vi "ziUpdateDevice.vi"(10 "file path (use dialog)":path=path "Z:/ziReleases/ci-artifacts/trunk/r49020-2017-11-30_15-47-53/LabOneMF-17.12.49020.tar", 11 "Address":string="DEV") -> (0 "Error Out":errorcluster)   [LabVIEW 2009, in "Zurich Instruments LabOne.lvlib"]
doc: "Allow to Update MFLI/UHF devices via the Labview API.\nNOTE: \nDO NOT TURN OFF POWER OR UNPLUG THE DEVICE FROM YOUR SYSTEM.PLEASE, WAIT UNTIL THE DEVICE IS FINISHED."
uses:
  <instrlib>/Zurich Instruments LabOne/Zurich Instruments LabOne.lvlib
  <instrlib>/Zurich Instruments LabOne/Public/Configure/ziGetValueString.vi
  <instrlib>/Zurich Instruments LabOne/Public/Configure/ziSetValueDouble.vi
  <instrlib>/Zurich Instruments LabOne/Public/Data/ziTypeCoreVectorWave.ctl
  <instrlib>/Zurich Instruments LabOne/Public/Configure/ziSetVector.vi
  <instrlib>/Zurich Instruments LabOne/Private/ziLV32.dll
panel:
  # "NOTE: \nDO NOT TURN OFF POWER OR UNPLUG \nTHE DEVICE FROM YOUR SYSTEM.\nPLEASE, WAIT UNTIL THE DEVICE IS FINISHED."
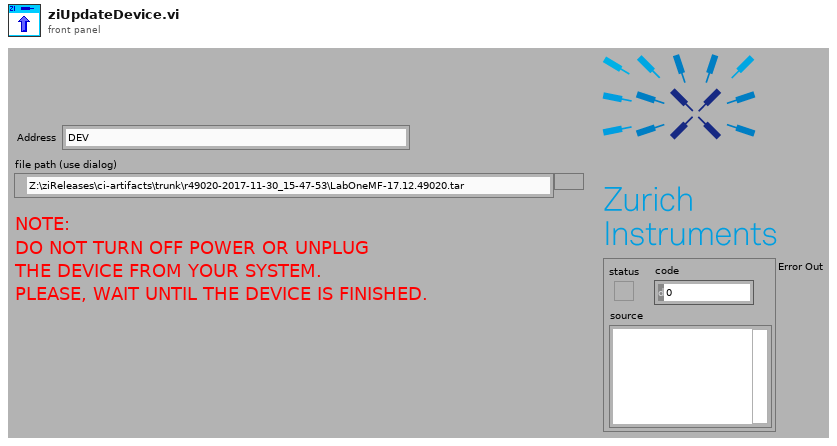
[diagram p1: front panel]
types:
  T1 = typedef "Zurich Instruments LabOne.lvlib/ziTypeCoreVectorWave.ctl" = cluster{"Timestamp (ticks)":u64, "Sequence Number":u32, "total Elements":u64, "Block Offset":u64, "Block Elements":u32, "Flags":u8, "Element Type":u8, "Data UInt8":u8[], "Data UInt16":u16[], "Data UInt32":u32[], "Data UInt64":u64[], "Data Float":sgl[], "Data Double":dbl[], "Data String":string}
  T2 = typedef "Zurich Instruments LabOne.lvlib/ziTypeHandle.ctl" = cluster{"handleValid":bool, "Conn":u64, "Path Prefix":string, "Handle":u64, "Connected":bool, "Clockbase(s)":dbl}
  T3 = typedef "ziTypeDisovery.ctl" = cluster{"timestamp":u64, "deviceid":string, "devicetype":string, "serveraddress":string, "serverport":u32, "apilevel":u32, "discoverable":bool, "interface":string, "connected":string, "available":bool, "owner":string, "status":string, "options ":string, "serverversion":string}
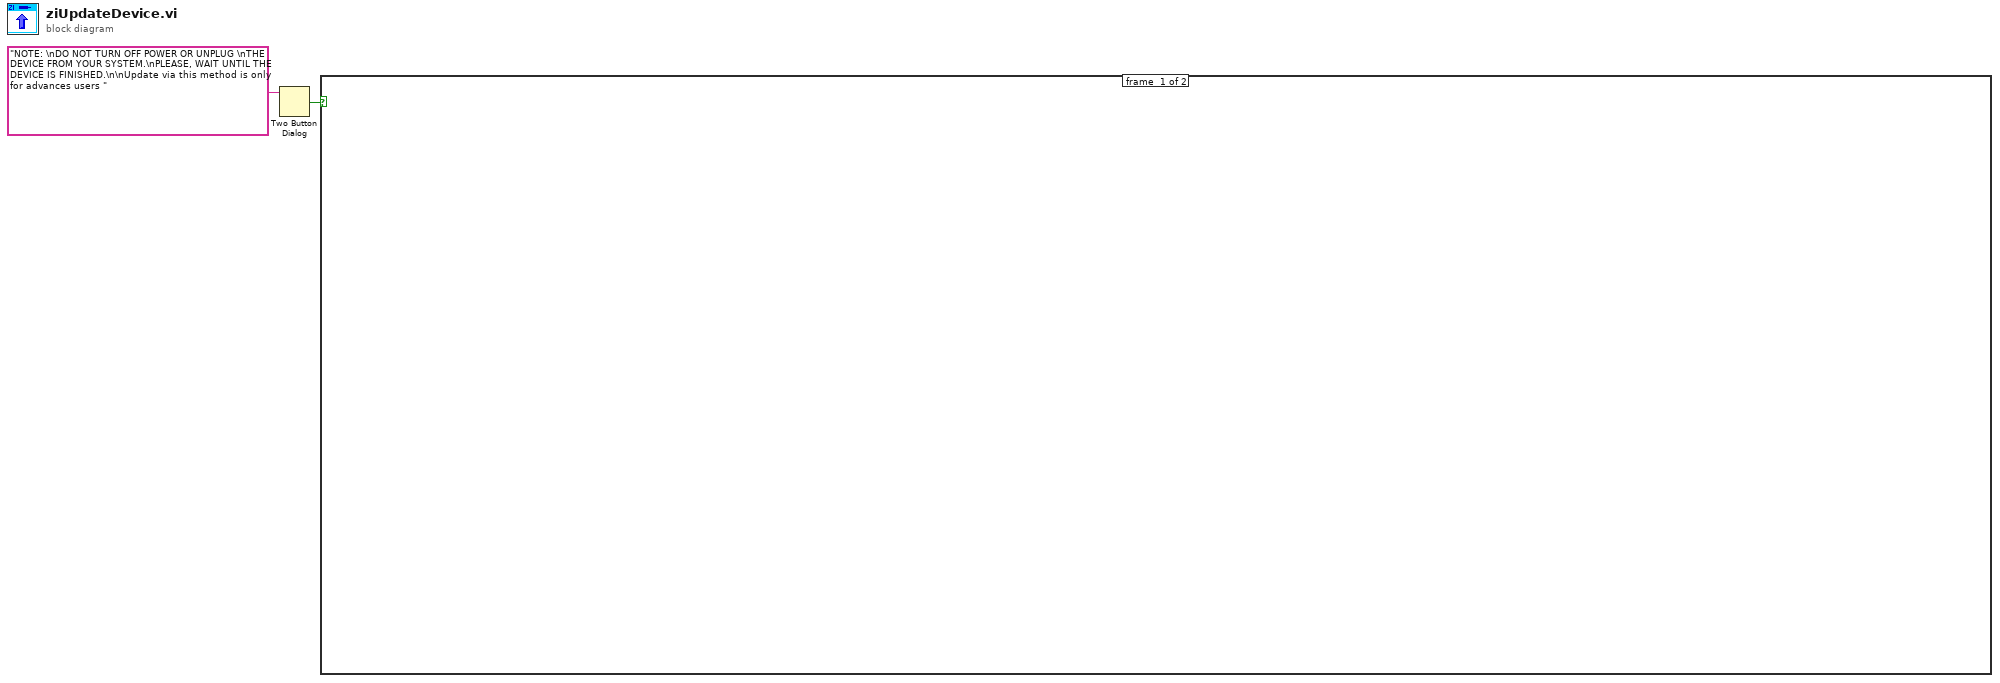
[diagram p0: block diagram]
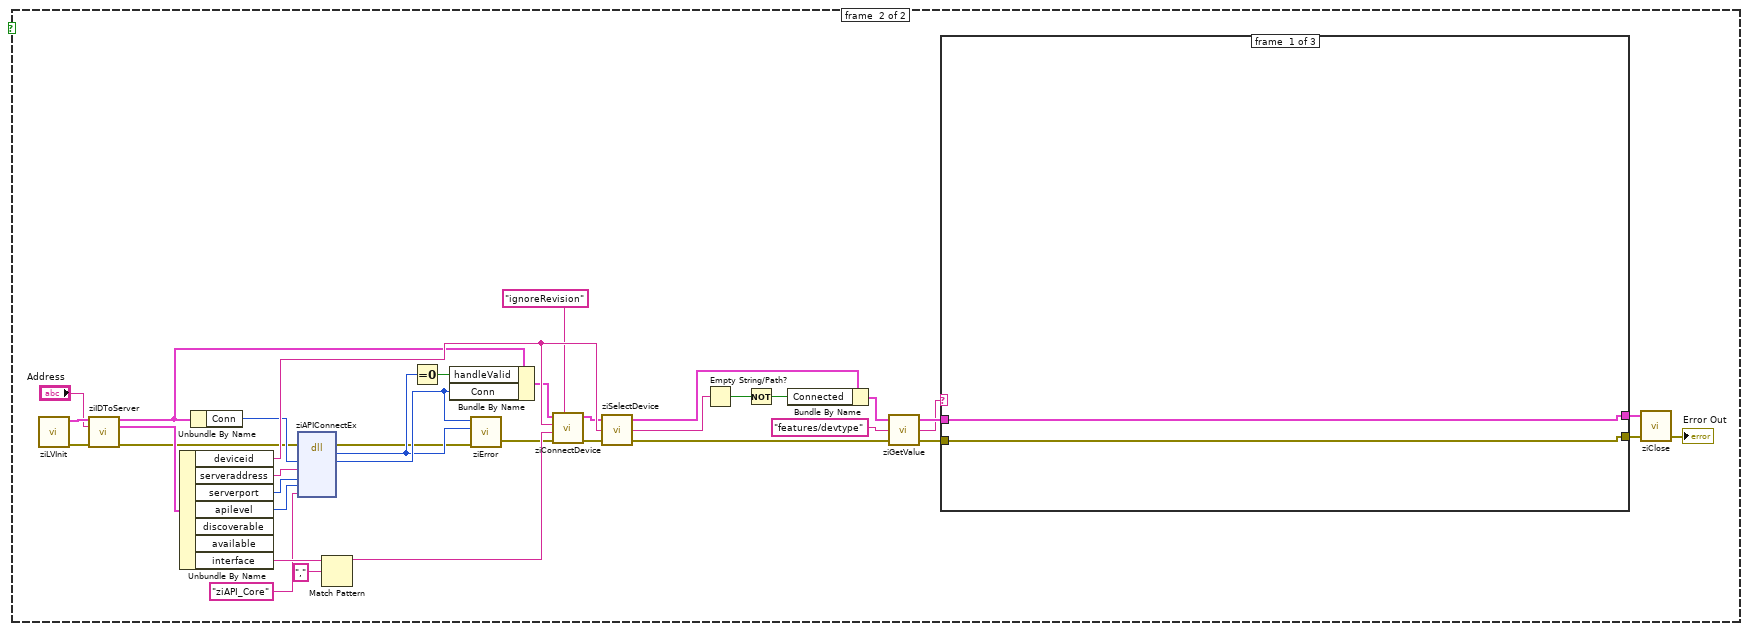
[diagram p2: hidden frame]
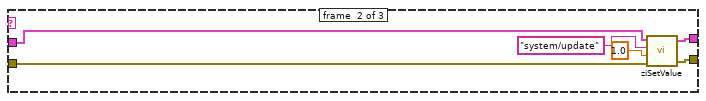
[diagram p3: hidden frame]
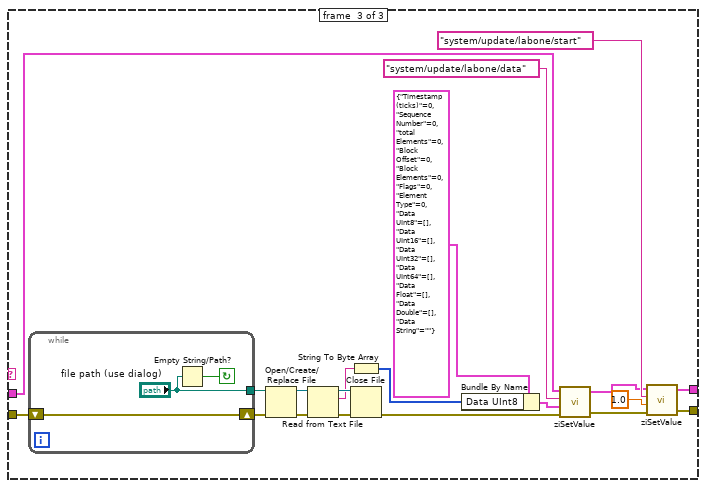
[diagram p4: hidden frame]
diagram:
  n1 = Two Button Dialog(message="NOTE: \nDO NOT TURN OFF POWER OR UNPLUG \nTHE DEVICE FROM YOUR SYSTEM.\nPLEASE, WAIT UNTIL THE DEVICE IS FINISHED.\n\nUpdate via this method is only for advances users ") -> (T button?=w1:bool)  [unwired: 2 in]
  n2 = case shown="True" w1 {
    frame #0 {
    }
    frame #1 {
      n3 = call <instrlib>:"ziLVInit.vi"() -> ("Error Out"=w14:errorcluster, "ziHandle"=w15:T2)  [unwired: 10 in]
      n4 = call <instrlib>:"ziIDToServer.vi"("ziHandle In"=w15, "Device ID"="Address", "Error In"=w14) -> ("ziHandle Out"=w12:T2, "ziDiscovery"=w11:T3, "Error Out"=w10:errorcluster)  [unwired: 10 in]
      n5 = Unbundle By Name(w11) -> ("deviceid"=w29:string, "serveraddress"=w19:string, "serverport"=w20:u32, "apilevel"=w21:u32, "interface"=w30:string)  [unwired: 2 out]
      n6 = Unbundle By Name(w12) -> ("Conn"=w22:u64)
      n7 = dll-call lib="C:/Program Files (x86)/National Instruments/LabVIEW 2009/instr.lib/Zurich Instruments LabOne/Private/ziLV*.*" fn="ziAPIConnectEx"(error in=w10, "Conn"=w22, "hostname"=w19, "Port"=w20, "ZIAPIVersion_enum"=w21, "Implementation"="ziAPI_Core") -> (error out=w16:errorcluster, "return type"=w17:u32, "Conn"=w23:u64)  [unwired: 6 in, 1 out]
      n8 = Match Pattern(string=w30, regular expression="," ("replace string (\"\")")) -> (before substring=w31:string)  [unwired: 1 in, 3 out]
      n9 = Equal To 0?(x=w17) -> (x = 0?=w24:bool)
      n10 = Bundle By Name(cluster=w12, "handleValid"=w24, "Conn"=w23) -> (w13:T2)
      n11 = call <instrlib>:"ziError.vi"("Conn"=w23, "ziErrorCode"=w17, "Error In"=w16) -> ("Error Out"=w9:errorcluster)  [unwired: 3 in]
      n12 = call <instrlib>:"ziConnectDevice.vi"("Device Interface Params (\"\")"="ignoreRevision" ("Device Interface Params (\"\")"), "Error In"=w9, "Device Interface"=w31, "Device Serial"=w29, "Handle In"=w13) -> ("Error Out"=w8:errorcluster, "Handle Out"=w7:T2)  [unwired: 5 in]
      n13 = call <instrlib>:"ziSelectDevice.vi"("Error In"=w8, "Device (first)"=w29, "Handle In"=w7) -> ("Error Out"=w5:errorcluster, "Selected Device"=w26:string, "Handle Out"=w25:T2)
      n14 = Empty String/Path?(string/path=w26) -> (empty?=w27:bool)
      n15 = Not(x=w27) -> (.not. x?=w28:bool)
      n16 = Bundle By Name(cluster=w25, "Connected"=w28) -> (w6:T2)
      n17 = call-poly <instrlib>:"ziGetValue.vi"("error in"=w5, "Path"="features/devtype", "Handle In"=w6) -> ("error out"=w38:errorcluster, "Value"=w36:string, "Handle Out"=w39:T2)
      n18 = case shown="Default" w36 {
        tunnel: w39 -> [w40 w47 w67]
        tunnel: w38 -> [w41 w46 w60]
        tunnel: [w40 w44 w49] -> w35
        tunnel: [w41 w45 w48] -> w34
        frame #0 {
        }
        frame #1 {
          n19 = call-poly <instrlib>:"ziSetValue.vi"("Error In"=w46, "Value"=1.0, "Path"="system/update", "Handle In"=w47) -> ("Error Out"=w45:errorcluster, "Handle Out"=w44:T2)  [unwired: 1 in]
        }
        frame #2 {
          n20 = while {
            tunnel: ["file path (use dialog)"] -> w63
            shift-right: [w68] -> w59
            shift-left: w60 -> [w68]
            stop <- w69 continue-if-true
            n21 = Empty String/Path?(string/path="file path (use dialog)") -> (empty?=w69:bool)
          }
          n22 = Open/Create/Replace File(file path (use dialog)=w63, error in=w59) -> (refnum out=w55:refnum<file>, error out=w54:errorcluster)  [unwired: 4 in, 1 out]
          n23 = Read from Text File(file (use dialog)=w55, error in=w54) -> (refnum out=w52:refnum<file>, text=w51:string, error out=w53:errorcluster)  [unwired: 2 in, 1 out]
          n24 = String To Byte Array(string=w51) -> (unsigned byte array=w50:u8[])
          n25 = Close File(refnum=w52, error in=w53) -> (error out=w64:errorcluster)  [unwired: 1 out]
          n26 = Bundle By Name(cluster=T1 {"Timestamp (ticks)"=0, "Sequence Number"=0, "total Elements"=0, "Block Offset"=0, "Block Elements"=0, "Flags"=0, "Element Type"=0, "Data UInt8"=[], "Data UInt16"=[], "Data UInt32"=[], "Data UInt64"=[], "Data Float"=[], "Data Double"=[], "Data String"=""} ("VectorWave In"), "Data UInt8"=w50) -> (w65:T1)
          n27 = call-poly <instrlib>:"ziSetValue.vi"("error in"=w64, "VectorWave In"=w65, "Path"="system/update/labone/data", "Handle in"=w67) -> ("error out"=w57:errorcluster, "Handle out"=w58:T2)  [unwired: 1 out]
          n28 = call-poly <instrlib>:"ziSetValue.vi"("Error In"=w57, "Value"=1.0, "Path"="system/update/labone/start", "Handle In"=w58) -> ("Error Out"=w48:errorcluster, "Handle Out"=w49:T2)  [unwired: 1 in]
        }
      }
      n29 = call <instrlib>:"ziClose.vi"("Error In"=w34, "Handle In"=w35) -> ("Error Out"=→"Error Out":errorcluster)  [unwired: 2 in, 1 out]
    }
  }
